vi "Reconstruct_STFT.vi"(5 "Group Number":i32, 6 "전체_Selected":i32[](array[numeric]), 7 "Selected":i32[](array[numeric]), 11 "STFT_CutOff":dbl[][](array[numeric])) -> (3 "STFT_FULL":dbl[][](array[numeric]))   [LabVIEW 2014]
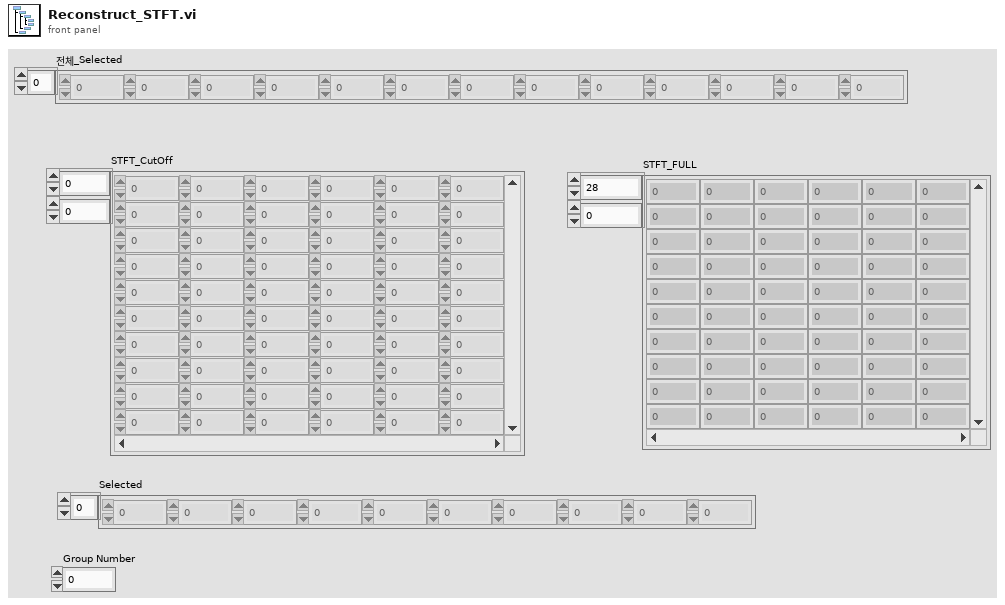
[diagram p1: front panel]
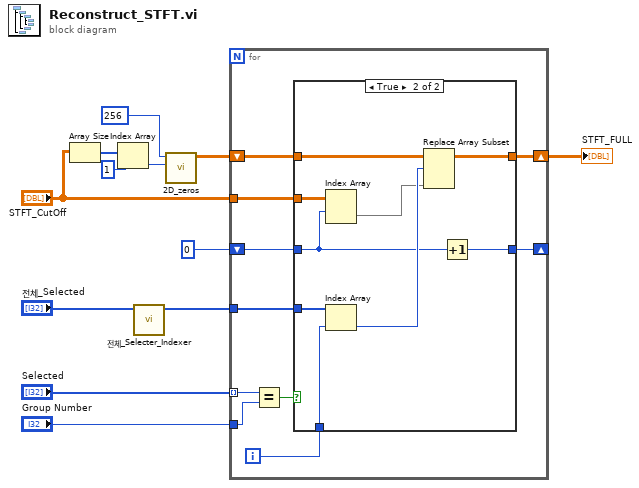
[diagram p0: block diagram]
diagram:
  n1 = Array Size(array="STFT_CutOff") -> (size(s)=w11:i32[])
  n2 = Index Array(array=w11, index=1) -> (element=w4:i32)
  n3 = call "전체_Selecter_Indexer.vi"("전체_Selected"="전체_Selected") -> ("Selected_Index"=w7:i32[])  [unwired: 10 in]
  n4 = call "2D_zeros.vi"("column_number"=w4, "row_number"=256 ("index")) -> ("2D_Rand"=w5:dbl[][])  [unwired: 9 in]
  n5 = for {
    tunnel: "Selected" -> [w22] mode=indexing
    tunnel: "STFT_CutOff" -> [w19]
    tunnel: "Group Number" -> [w21]
    tunnel: w7 -> [w17]
    shift-right: [w15] -> w2
    shift-left: w5 -> [w18]
    shift-right: [w13] -> _
    shift-left: 0 -> [w14]
    i -> [w16]
    n6 = Equal?(x=w22, y=w21) -> (x = y?=w20:bool)
    n7 = case shown="True" w20 {
      tunnel: w19 -> [_ w33]
      tunnel: w18 -> [w24 w31]
      tunnel: w17 -> [_ w32]
      tunnel: w16 -> [_ w27]
      tunnel: [w24 w28] -> w15
      tunnel: w14 -> [w23 w26]
      tunnel: [w23 w25] -> w13
      frame False {
      }
      frame True {
        n8 = Index Array(array=w33, index (row)=w26) -> (element=w29:dbl[])  [unwired: 1 in]
        n9 = Index Array(array=w32, index=w27) -> (element=w30:i32)
        n10 = Replace Array Subset(array=w31, new element=w29, index (row)=w30) -> (w28:dbl[][])  [unwired: 1 in]
        n11 = Increment(x=w26) -> (x+1=w25:i32)
      }
    }
  }
  "STFT_FULL" <- w2
